vi "写入测量参数.vi"(8 "error in (no error)":errorcluster caption="错误输入（无错误）", 10 "测量参数":T1(ring), 11 "数字多用表接口输入":refnum<class "数字多用表接口.lvclass">) -> (0 "error out":errorcluster caption="错误输出", 3 "数字多用表接口输出":refnum<class "数字多用表接口.lvclass">)   [LabVIEW 2020, in "数字多用表接口.lvlib" / "数字多用表接口.lvclass"]
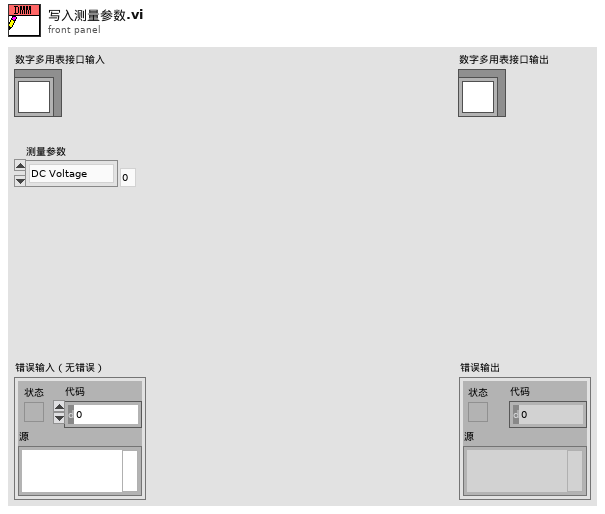
[diagram p1: front panel]
types:
  T1 = enum16{"DC Voltage", "AC Voltage", "Resistance", "DC Current", "AC Current"}
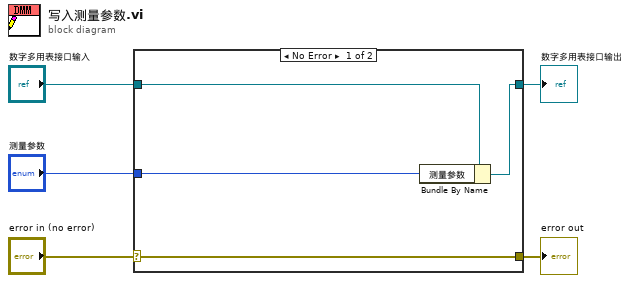
[diagram p0: block diagram]
diagram:
  n1 = case shown="No Error" "error in (no error)" {
    selector: "error in (no error)" -> [w9 w10]
    tunnel: [w9 w10] -> w4
    tunnel: [w7 w11] -> w2
    tunnel: "数字多用表接口输入" -> [w8 w11]
    tunnel: "测量参数" -> [w6 _]
    frame No Error {
      n2 = Bundle By Name(cluster=w8, "测量参数"=w6) -> (w7:refnum<class "数字多用表接口.lvclass">)
    }
    frame Error {
    }
  }
  "error out" <- w4
  "数字多用表接口输出" <- w2
